vi "Generator simplified.vi"(1 "ON (F)":bool) -> (0 "Q":bool)   [LabVIEW 2019, in "Counter.lvlib"]
uses:
  Counter.lvlib
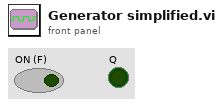
[diagram p1: front panel]
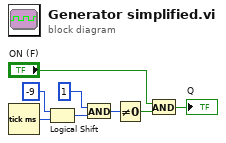
[diagram p0: block diagram]
diagram:
  n1 = Tick Count (ms)() -> (millisecond timer value=w2:u32)
  n2 = Logical Shift(y=i16 -9, x=w2) -> (x << y=w7:u32)
  n3 = And(x=u32 1 ("y"), y=w7) -> (x .and. y?=w5:u32)
  n4 = Not Equal To 0?(x=w5) -> (x != 0?=w4:bool)
  n5 = And(x="ON (F)", y=w4) -> (x .and. y?=→"Q":bool)
